vi "postion store.vi"(7 "R/W":enum16{"write", "read"}(ring), 10 "Write":T1[](array[typedef])) -> (2 "read":T1[](array[typedef]))   [LabVIEW 2019]
uses:
  ctl/position array.ctl
  ctl/position name.ctl
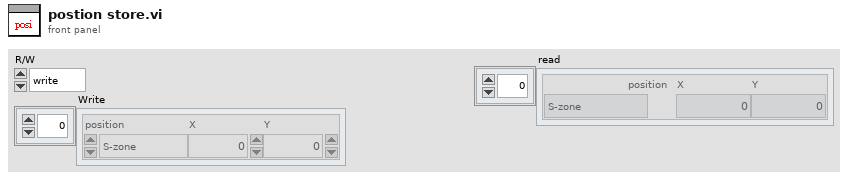
[diagram p1: front panel]
types:
  T1 = typedef "position array.ctl" = cluster{"position":T2, "X":dbl, "Y":dbl}
  T2 = typedef "position name.ctl" = enum16{"S-zone", "out S", "vision board-vision", "out box", "box catch", "room center", "room right", "room left", "R2", "R4", "only rotate", "out recy", "recycle", "R3", "near board", "box poxition", "R1", "R5", "R1-d", "R5-d", "R3.4", "align center.1", "align center.5", "R2-d", "R2-r", "far center"}
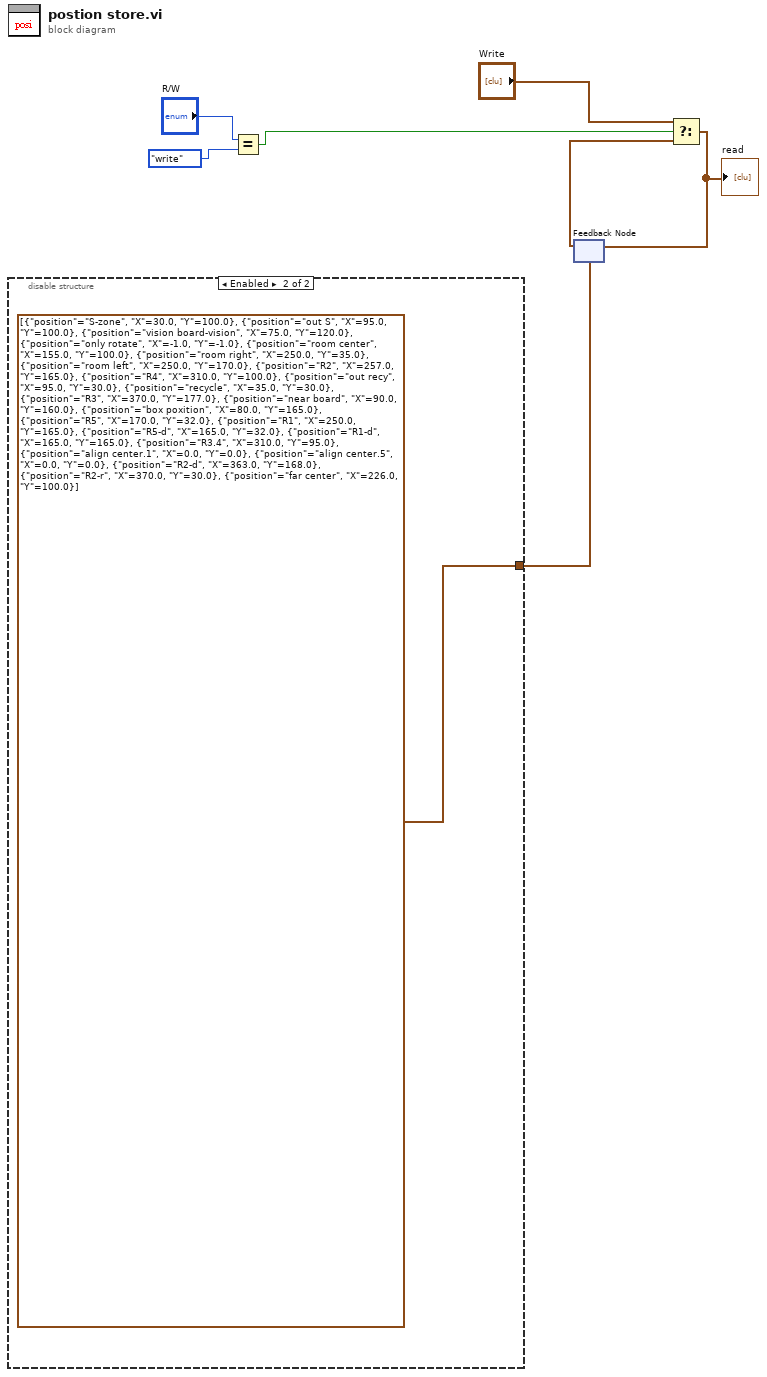
[diagram p0: block diagram]
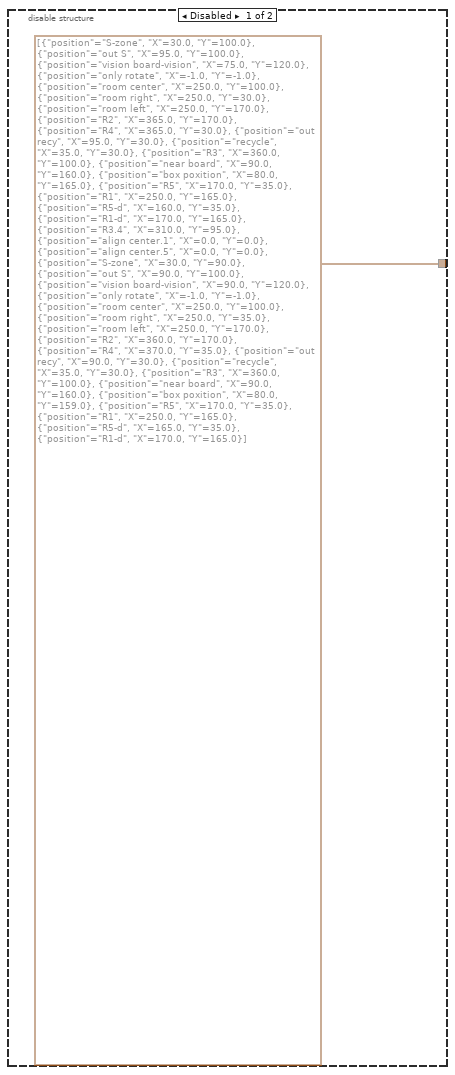
[diagram p2: hidden frame]
diagram:
  n1 = disable-structure shown="Enabled" {
    disable-tunnel: [T1[] [{"position"=enum."S-zone", "X"=30.0, "Y"=100.0}, {"position"=enum."out S", "X"=95.0, "Y"=100.0}, {"position"=enum."vision board-vision", "X"=75.0, "Y"=120.0}, {"position"=enum."only rotate", "X"=-1.0, "Y"=-1.0}, {"position"=enum."room center", "X"=250.0, "Y"=100.0}, {"position"=enum."room right", "X"=250.0, "Y"=30.0}, {"position"=enum."room left", "X"=250.0, "Y"=170.0}, {"position"=enum."R2", "X"=365.0, "Y"=170.0}, {"position"=enum."R4", "X"=365.0, "Y"=30.0}, {"position"=enum."out recy", "X"=95.0, "Y"=30.0}, {"position"=enum."recycle", "X"=35.0, "Y"=30.0}, {"position"=enum."R3", "X"=360.0, "Y"=100.0}, {"position"=enum."near board", "X"=90.0, "Y"=160.0}, {"position"=enum."box poxition", "X"=80.0, "Y"=165.0}, {"position"=enum."R5", "X"=170.0, "Y"=35.0}, {"position"=enum."R1", "X"=250.0, "Y"=165.0}, {"position"=enum."R5-d", "X"=160.0, "Y"=35.0}, {"position"=enum."R1-d", "X"=170.0, "Y"=165.0}, {"position"=enum."R3.4", "X"=310.0, "Y"=95.0}, {"position"=enum."align center.1", "X"=0.0, "Y"=0.0}, {"position"=enum."align center.5", "X"=0.0, "Y"=0.0}, {"position"=enum."S-zone", "X"=30.0, "Y"=90.0}, {"position"=enum."out S", "X"=90.0, "Y"=100.0}, {"position"=enum."vision board-vision", "X"=90.0, "Y"=120.0}, {"position"=enum."only rotate", "X"=-1.0, "Y"=-1.0}, {"position"=enum."room center", "X"=250.0, "Y"=100.0}, {"position"=enum."room right", "X"=250.0, "Y"=35.0}, {"position"=enum."room left", "X"=250.0, "Y"=170.0}, {"position"=enum."R2", "X"=360.0, "Y"=170.0}, {"position"=enum."R4", "X"=370.0, "Y"=35.0}, {"position"=enum."out recy", "X"=90.0, "Y"=30.0}, {"position"=enum."recycle", "X"=35.0, "Y"=30.0}, {"position"=enum."R3", "X"=360.0, "Y"=100.0}, {"position"=enum."near board", "X"=90.0, "Y"=160.0}, {"position"=enum."box poxition", "X"=80.0, "Y"=159.0}, {"position"=enum."R5", "X"=170.0, "Y"=35.0}, {"position"=enum."R1", "X"=250.0, "Y"=165.0}, {"position"=enum."R5-d", "X"=165.0, "Y"=35.0}, {"position"=enum."R1-d", "X"=170.0, "Y"=165.0}] ("Array") T1[] [{"position"=enum."S-zone", "X"=30.0, "Y"=100.0}, {"position"=enum."out S", "X"=95.0, "Y"=100.0}, {"position"=enum."vision board-vision", "X"=75.0, "Y"=120.0}, {"position"=enum."only rotate", "X"=-1.0, "Y"=-1.0}, {"position"=enum."room center", "X"=155.0, "Y"=100.0}, {"position"=enum."room right", "X"=250.0, "Y"=35.0}, {"position"=enum."room left", "X"=250.0, "Y"=170.0}, {"position"=enum."R2", "X"=257.0, "Y"=165.0}, {"position"=enum."R4", "X"=310.0, "Y"=100.0}, {"position"=enum."out recy", "X"=95.0, "Y"=30.0}, {"position"=enum."recycle", "X"=35.0, "Y"=30.0}, {"position"=enum."R3", "X"=370.0, "Y"=177.0}, {"position"=enum."near board", "X"=90.0, "Y"=160.0}, {"position"=enum."box poxition", "X"=80.0, "Y"=165.0}, {"position"=enum."R5", "X"=170.0, "Y"=32.0}, {"position"=enum."R1", "X"=250.0, "Y"=165.0}, {"position"=enum."R5-d", "X"=165.0, "Y"=32.0}, {"position"=enum."R1-d", "X"=165.0, "Y"=165.0}, {"position"=enum."R3.4", "X"=310.0, "Y"=95.0}, {"position"=enum."align center.1", "X"=0.0, "Y"=0.0}, {"position"=enum."align center.5", "X"=0.0, "Y"=0.0}, {"position"=enum."R2-d", "X"=363.0, "Y"=168.0}, {"position"=enum."R2-r", "X"=370.0, "Y"=30.0}, {"position"=enum."far center", "X"=226.0, "Y"=100.0}] ("Array")] -> w7
    frame Disabled {
    }
    frame Enabled {
    }
  }
  n2 = Equal?(x="R/W", y=enum16{"write", "read"}."write" ("R/W")) -> (x = y?=w4:bool)
  n3 = feedback #1(w7) -> (w2:T1[])
  n4 = Select(t="Write", s=w4, f=w2) -> (s? t:f=w3:T1[])
  "read" <- w3
  n5 = feedback-in #1(w3) -> ()
